vi "Local Search_IRH3T Best Solution.vi"(8 "error in (no error)":errorcluster, 10 "OSSP_Problem in":refnum<class "OSSP_Problem.lvclass">, 11 "GA in":refnum<class "GA.lvclass">) -> (0 "error out":errorcluster, 2 "OSSP_Problem out":refnum<class "OSSP_Problem.lvclass">, 3 "GA out":refnum<class "GA.lvclass">)   [LabVIEW 2013]
uses:
  Classes/GA.lvclass
  Classes/OSSP_Problem.lvclass
  Classes/OSSP_Problem.lvclass/OSSP_Problem.ctl
  Classes/GA.lvclass/GA.ctl
  Classes/Scheduler_Class/NonDelay Scheduler/Non Delay Scheduler Engine.vi
  GA/SubVIS/Calcualte General Tardiness.vi
  Classes/Scheduler_Class/Operation to Machine Job Tuple.vi
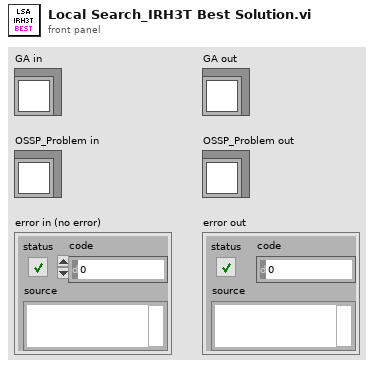
[diagram p1: front panel]
types:
  T1 = typedef "Solution_GA.ctl" = cluster{"Schedule":u16[], "Fitness":u16, "Fitness Valid?":bool}
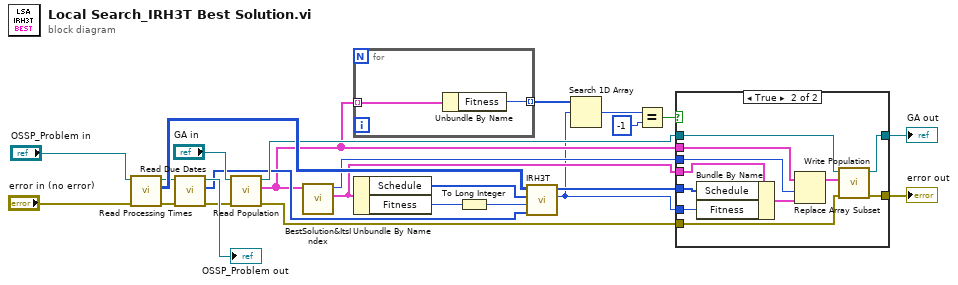
[diagram p0: block diagram]
diagram:
  n1 = call "Read Processing Times.vi"("error in (no error)"="error in (no error)", "OSSP_Problem in"="OSSP_Problem in") -> ("error out"=w17:errorcluster, "Processing Times"=w19:u16[][], "OSSP_Problem out"=w18:refnum<class "OSSP_Problem.lvclass">)  [unwired: 7 in]
  n2 = call "Read Due Dates.vi"("error in (no error)"=w17, "OSSP_Problem in"=w18) -> ("error out"=w16:errorcluster, "Due Dates"=w7:u16[], "OSSP_Problem out"=→"OSSP_Problem out":refnum<class "OSSP_Problem.lvclass">)  [unwired: 7 in]
  n3 = call "Read Population.vi"("error in (no error)"=w16, "GA in"="GA in") -> ("error out"=w14:errorcluster, "Population"=w6:T1[], "GA out"=w15:refnum<class "GA.lvclass">)  [unwired: 7 in]
  n4 = call "BestSolution&ItsIndex.vi"("Population"=w6) -> ("Best Solution In the Population"=w12:T1, "Best Solution Index for Replace"=w11:i32)  [unwired: 9 in]
  n5 = for {
    tunnel: w6 -> [w27] mode=indexing
    tunnel: [w26] -> w5 mode=indexing
    n6 = Unbundle By Name(w27) -> ("Fitness"=w26:u16)
  }
  n7 = Unbundle By Name(w12) -> ("Schedule"=w10:u16[], "Fitness"=w9:u16)
  n8 = To Long Integer(number=w9) -> (32bit integer=w8:i32)
  n9 = call "IRH3T.vi"("Due Dates"=w7, "Initial Tardiness"=w8, "Schedule 2B Improved"=w10, "Proocessing Times  (Machines x Jobs)"=w19) -> ("Total Tardiness"=w4:u16, "IRH3T (Reordered) Schedule Out"=w13:u16[])  [unwired: 5 in, 1 out]
  n10 = Search 1D Array(1D array=w5, element=w4) -> (index of element=w3:i32)  [unwired: 1 in]
  n11 = Equal?(x=w3, y=-1) -> (x = y?=w1:bool)
  n12 = case shown="True" w1 {
    tunnel: w15 -> [w28 w40]
    tunnel: w14 -> [w29 w39]
    tunnel: [w29 w38] -> w23
    tunnel: w13 -> [_ w37]
    tunnel: [w28 w36] -> w25
    tunnel: w12 -> [_ w35]
    tunnel: w11 -> [_ w34]
    tunnel: w6 -> [_ w31]
    tunnel: w4 -> [_ w30]
    frame False {
    }
    frame True {
      n13 = Bundle By Name(cluster=w35, "Schedule"=w37, "Fitness"=w30) -> (w33:T1)
      n14 = Replace Array Subset(array=w31, new element=w33, index=w34) -> (w32:T1[])
      n15 = call "Write Population.vi"("error in (no error)"=w39, "Population"=w32, "GA in"=w40) -> ("error out"=w38:errorcluster, "GA out"=w36:refnum<class "GA.lvclass">)  [unwired: 7 in]
    }
  }
  "GA out" <- w25
  "error out" <- w23
